vi "3D-Param Collect.vi"(8 "New Array":string[](array[string]), 10 "ColNumber":i32, 11 "Test Result":string[][](table)) -> (3 "Test Result 2":string[][](table))   [LabVIEW 2011]
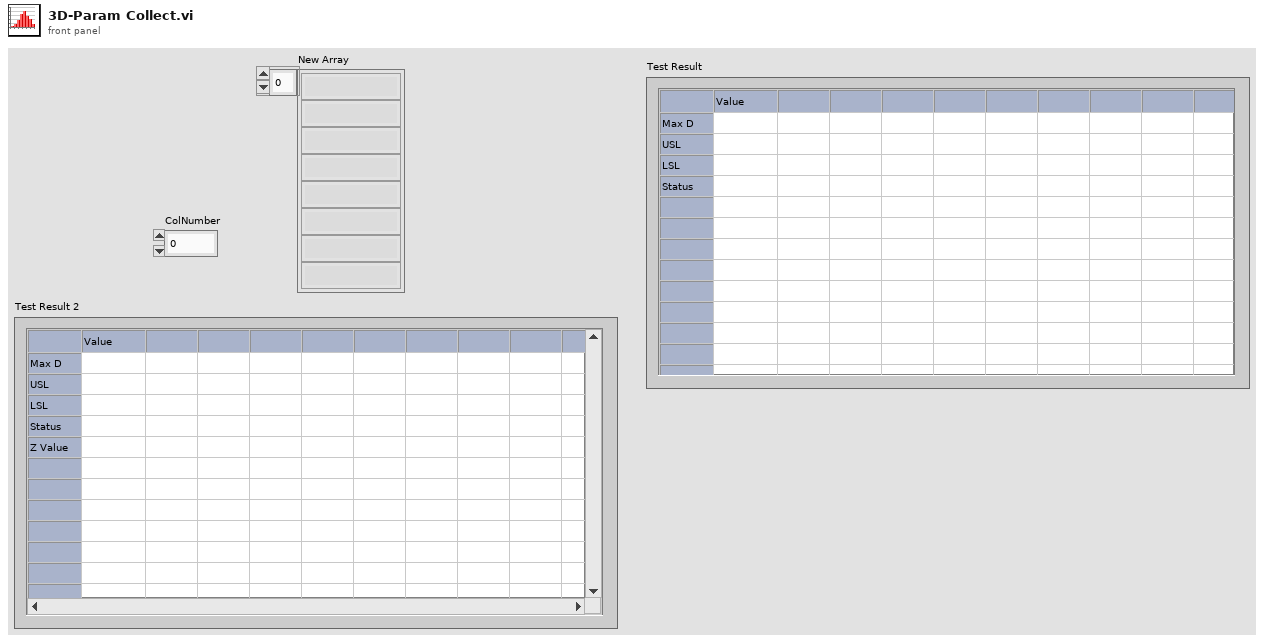
[diagram p1: front panel]
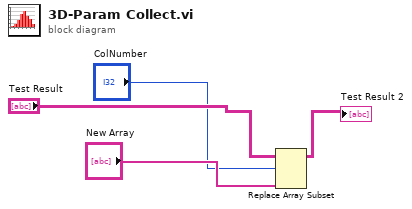
[diagram p0: block diagram]
diagram:
  n1 = Replace Array Subset(array="Test Result", new element="New Array", index (row)="ColNumber") -> (→"Test Result 2":string[][])  [unwired: 1 in]
